vi "Create Message Queue.vi"(8 "error in (no error)":errorcluster, 11 "queue name":string) -> (0 "error out":errorcluster, 3 "Message queue":refnum<queue>)   [LabVIEW 2021]
uses:
  Message.ctl
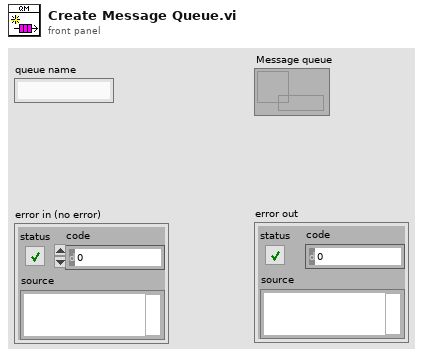
[diagram p1: front panel]
types:
  T1 = typedef "Message.ctl" = cluster{"Name":string, "Value":string, "Local IP":string, "Local Queue":string, "Remote IP":string, "Remote Queue":string}
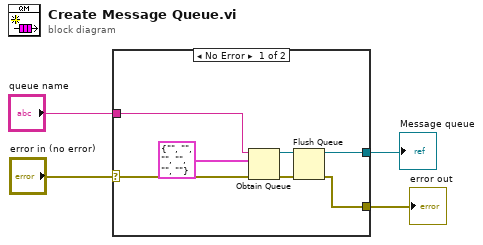
[diagram p0: block diagram]
diagram:
  n1 = case shown="No Error" "error in (no error)" {
    selector: "error in (no error)" -> [w9 w12]
    tunnel: "queue name" -> [w8 _]
    tunnel: [w11 w12] -> w3
    tunnel: [w10 _] -> w1
    frame No Error {
      n2 = Obtain Queue(name (unnamed)=w8, element data type=T1 {"Name"="", "Value"="", "Local IP"="", "Local Queue"="", "Remote IP"="", "Remote Queue"=""} ("Message"), error in (no error)=w9) -> (queue out=w7:refnum<queue>, error out=w6:errorcluster)  [unwired: 2 in, 1 out]
      n3 = Flush Queue(queue=w7, error in (no error)=w6) -> (queue out=w10:refnum<queue>, error out=w11:errorcluster)  [unwired: 1 out]
    }
    frame Error {
    }
  }
  "error out" <- w3
  "Message queue" <- w1
